vi "kzstc.vi"(9 "触发时间输入":i32 caption="mS", 10 "NewVal":bool, 11 "定时":bool) -> (2 "触发时间输出":i32, 3 "禁用":T1(ring))   [LabVIEW 2012]
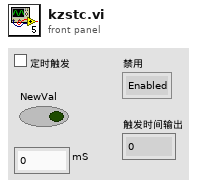
[diagram p1: front panel]
types:
  T1 = enum8{"Enabled", "Disabled", "Disabled and Grayed Out"}
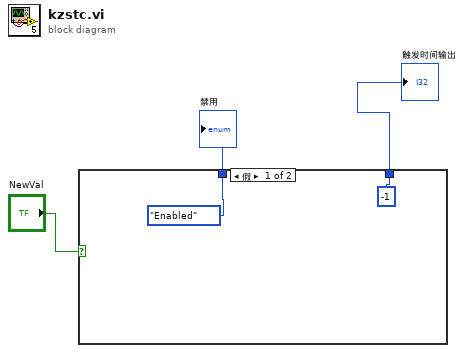
[diagram p0: block diagram]
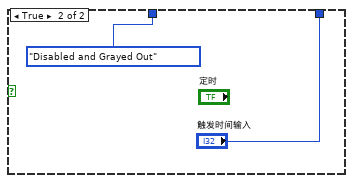
[diagram p2: hidden frame]
diagram:
  n1 = case shown="假" "NewVal" {
    tunnel: [-1 ("触发时间") "触发时间输入"] -> w1
    tunnel: [T1."Enabled" ("禁用") T1."Disabled and Grayed Out" ("禁用")] -> w3
    frame False {
    }
    frame True {
    }
  }
  "禁用" <- w3
  "触发时间输出" <- w1
